vi "Write Compression_.vi"(8 "error in (no error)":errorcluster, 10 "Compression?":bool, 11 "Servo MSMT in":refnum<class "Servo MSMT.lvclass">) -> (0 "error out":errorcluster, 3 "Servo MSMT out":refnum<class "Servo MSMT.lvclass">)   [LabVIEW 2018, in "Servo MSMT.lvlib" / "Servo MSMT.lvclass"]
uses:
  Servo MSMT.lvclass
  Servo MSMT.lvclass/Servo MSMT.ctl
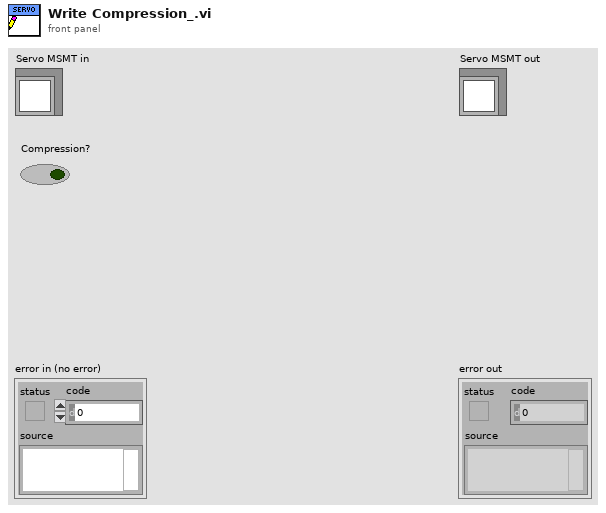
[diagram p1: front panel]
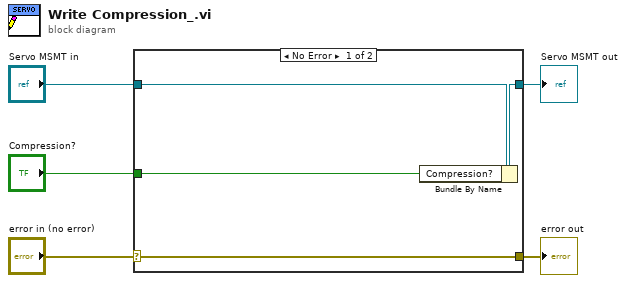
[diagram p0: block diagram]
diagram:
  n1 = case shown="No Error" "error in (no error)" {
    selector: "error in (no error)" -> [w9 w10]
    tunnel: [w9 w10] -> w4
    tunnel: [w7 w11] -> w2
    tunnel: "Servo MSMT in" -> [w8 w11]
    tunnel: "Compression?" -> [w6 _]
    frame No Error {
      n2 = Bundle By Name(cluster=w8, "Compression?"=w6) -> (w7:refnum<class "Servo MSMT.lvclass">)
    }
    frame Error {
    }
  }
  "error out" <- w4
  "Servo MSMT out" <- w2
